vi "Receive.vi"(6 "clear_timeout_error (f)":bool, 7 "mode (standard)":T1(ring), 8 "error in (no error)":errorcluster, 10 "bufsize (0)":u32, 11 "Socket.Base in":refnum<class "Socket.Base.lvclass">) -> (0 "error out":errorcluster, 1 "bytes_read":i32, 2 "data_out":string, 3 "Socket.Base out":refnum<class "Socket.Base.lvclass">)   [LabVIEW 2014, in "Socket.lvlib" / "Socket.Base.lvclass"]
doc: "(Must be Overridden.) Waits for the timeout period in ms and returns bytes received or timeout error. See the individual child classes for the input parameter usage"
uses:
  Socket.Base.lvclass
  <vilib>/Utility/error.llb/Error Cluster From Error Code.vi
  <vilib>/ErrorRing/Error Ring.xnode
panel:
  # "If bufsize is 0, a TCP packet is assumed and the first two bytes will be used as the packet size."
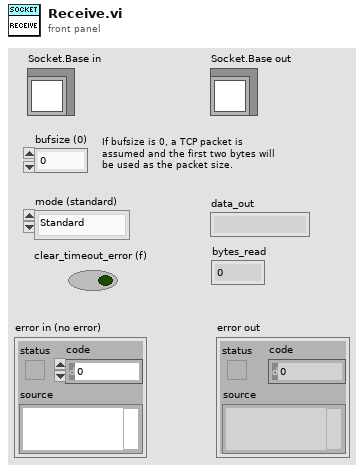
[diagram p1: front panel]
types:
  T1 = enum16{"Standard", "Buffered", "CRLF", "Immediate"}
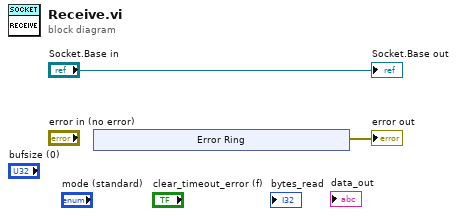
[diagram p0: block diagram]
diagram:
  n1 = xnode "Error Ring"() -> ("error out"=→"error out":errorcluster)
  "Socket.Base out" <- "Socket.Base in"
